vi "VoltageRatioInputStart.vi"(0 "Device Info":T1={"Serial Number"=-1, "Channel"=0, "Port"=0}, 1 "Data Interval":i32=-1, 2 "Change Trigger":dbl, 3 "Sesnor Type":u32(ring) caption="Sensor Type" items=["SENSOR_TYPE_VOLTAGERATIO"=0, "SENSOR_TYPE_1101_SHARP_2D120X"=11011, "SENSOR_TYPE_1101_SHARP_2Y0A21"=11012, "SENSOR_TYPE_1101_SHARP_2Y0A02"=11013, "SENSOR_TYPE_1102"=11020, "SENSOR_TYPE_1103"=11030, "SENSOR_TYPE_1104"=11040, "SENSOR_TYPE_1105"=11050, "SENSOR_TYPE_1106"=11060, "SENSOR_TYPE_1107"=11070, "SENSOR_TYPE_1108"=11080, "SENSOR_TYPE_1109"=11090, "SENSOR_TYPE_1110"=11100, "SENSOR_TYPE_1111"=11110, "SENSOR_TYPE_1112"=11120, "SENSOR_TYPE_1113"=11130, "SENSOR_TYPE_1115"=11150, "SENSOR_TYPE_1116"=11160, "SENSOR_TYPE_1118_AC"=11181, "SENSOR_TYPE_1118_DC"=11182, "SENSOR_TYPE_1119_AC"=11191, "SENSOR_TYPE_1119_DC"=11192, "SENSOR_TYPE_1120"=11200, "SENSOR_TYPE_1121"=11210, "SENSOR_TYPE_1122_AC"=11221, "SENSOR_TYPE_1122_DC"=11222, "SENSOR_TYPE_1124"=11240, "SENSOR_TYPE_1125_HUMIDITY"=11251, "SENSOR_TYPE_1125_TEMPERATURE"=11252, "SENSOR_TYPE_1126"=11260, "SENSOR_TYPE_1128"=11280, "SENSOR_TYPE_1129"=11290, "SENSOR_TYPE_1131"=11310, "SENSOR_TYPE_1134"=11340, "SENSOR_TYPE_1136"=11360, "SENSOR_TYPE_1137"=11370, "SENSOR_TYPE_1138"=11380, "SENSOR_TYPE_1139"=11390, "SENSOR_TYPE_1140"=11400, "SENSOR_TYPE_1141"=11410, "SENSOR_TYPE_1146"=11460, "SENSOR_TYPE_3120"=31200, "SENSOR_TYPE_3121"=31210, "SENSOR_TYPE_3122"=31220, "SENSOR_TYPE_3123"=31230, "SENSOR_TYPE_3130"=31300, "SENSOR_TYPE_3520"=35200, "SENSOR_TYPE_3521"=35210, "SENSOR_TYPE_3522"=35220], 5 "IsHubPort":bool, 7 "Bridge Enabled":bool=TRUE, 9 "Bridge Gain":u32(ring)=8 items=["BRIDGE_GAIN_1"=1, "BRIDGE_GAIN_2"=2, "BRIDGE_GAIN_4"=3, "BRIDGE_GAIN_8"=4, "BRIDGE_GAIN_16"=5, "BRIDGE_GAIN_32"=6, "BRIDGE_GAIN_64"=7, "BRIDGE_GAIN_128"=8], 11 "error in (no error)":errorcluster, 12 "Connection":u16(ring) items=["No Preference", "Remote", "Local"], 13 "Timeout (mSec)":i32=5000) -> (4 "Phidget ID":u64, 6 "Serial Number Return":i32, 10 "Attached?":bool, 15 "error out":errorcluster)   [LabVIEW 2012, in "Phidget Voltage Ratio Input.lvlib"]
doc: "${VoltageRatioInput:StartHeader}"
uses:
  <instrlib>/Phidgets/Phidget Voltage Ratio Input/Phidget Voltage Ratio Input.lvlib
  <instrlib>/Phidgets/Phidget Common/Phidget Common.lvlib
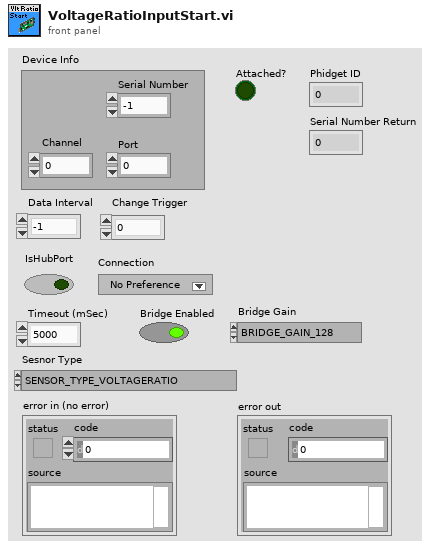
[diagram p1: front panel]
types:
  T1 = cluster{"Serial Number":i32, "Channel":i32, "Port":i32}
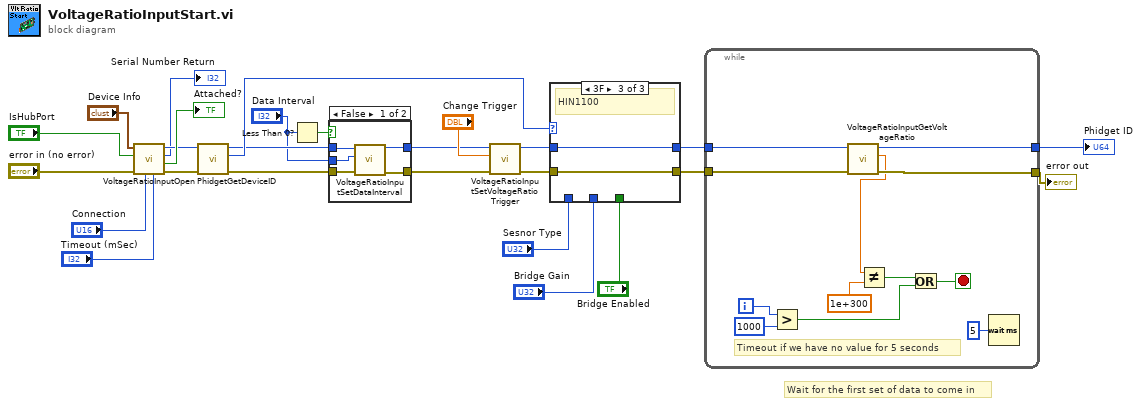
[diagram p0: block diagram]
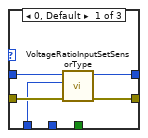
[diagram p3: hidden frame]
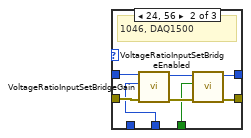
[diagram p4: hidden frame]
diagram:
  # "Wait for the first set of data to come in"
  n1 = call <instrlib>:"VoltageRatioInputOpen.vi"("Timeout (mSec)"="Timeout (mSec)", "Connection"="Connection", "error in"="error in (no error)", "IsHubPort"="IsHubPort", "Device Info"="Device Info") -> ("error out"=w23:errorcluster, "Attached?"=→"Attached?":bool, "Serial Number Return"=→"Serial Number Return":i32, "Phidget ID"=w22:u64)  [unwired: 3 in]
  n2 = call <instrlib>:"PhidgetGetDeviceID.vi"("error in (no error)"=w23, "Device In"=w22) -> ("error out"=w5:errorcluster, "Devie IDs"=w10:u32, "Device Out"=w4:u64)  [unwired: 6 in]
  n3 = Less Than 0?(x="Data Interval") -> (x < 0?=w6:bool)
  n4 = case shown="False" w6 {
    tunnel: w4 -> [w31 w33]
    tunnel: w5 -> [w30 w32]
    tunnel: [w28 w33] -> w2
    tunnel: [w29 w32] -> w1
    tunnel: "Data Interval" -> [w27 _]
    frame False {
      n5 = call <instrlib>:"VoltageRatioInputSetDataInterval.vi"("error in (no error)"=w30, "Interval"=w27, "Device In"=w31) -> ("error out"=w29:errorcluster, "Device Out"=w28:u64)  [unwired: 6 in]
    }
    frame True {
    }
  }
  n6 = call <instrlib>:"VoltageRatioInputSetVoltageRatioTrigger.vi"("error in (no error)"=w1, "Trigger"="Change Trigger", "Device In"=w2) -> ("error out"=w14:errorcluster, "Device Out"=w13:u64)  [unwired: 6 in]
  n7 = case shown="3F" w10 {
    tunnel: w14 -> [w38 w42 w47]
    tunnel: w13 -> [w37 w41 w48]
    tunnel: [w36 w43 w47] -> w12
    tunnel: [w35 w44 w48] -> w11
    tunnel: "Sesnor Type" -> [w34 _ _]
    tunnel: "Bridge Gain" -> [_ w40 _]
    tunnel: "Bridge Enabled" -> [_ w39 _]
    frame 0, Default {
      n8 = call <instrlib>:"VoltageRatioInputSetSensorType.vi"("error in (no error)"=w38, "Sesnor Type"=w34, "Device In"=w37) -> ("error out"=w36:errorcluster, "Device Out"=w35:u64)  [unwired: 6 in]
    }
    frame 24, 56 {
      # "1046, DAQ1500"
      n9 = call <instrlib>:"VoltageRatioInputSetBridgeGain.vi"("error in (no error)"=w42, "Bridge Gain"=w40, "Device In"=w41) -> ("error out"=w45:errorcluster, "Device Out"=w46:u64)  [unwired: 6 in]
      n10 = call <instrlib>:"VoltageRatioInputSetBridgeEnabled.vi"("error in (no error)"=w45, "Bridge Enabled"=w39, "Device In"=w46) -> ("error out"=w43:errorcluster, "Device Out"=w44:u64)  [unwired: 6 in]
    }
    frame 63 {
      # "HIN1100"
    }
  }
  n11 = while {
    tunnel: w11 -> [w58]
    tunnel: w12 -> [w57]
    tunnel: [w55] -> w21
    tunnel: [w56] -> w25
    i -> [w53]
    stop <- w50 stop-if-true
    # "Timeout if we have no value for 5 seconds"
    n12 = Greater?(x=w53, y=1000) -> (0:w51:bool)
    n13 = call <instrlib>:"VoltageRatioInputGetVoltageRatio.vi"("error in (no error)"=w57, "Device In"=w58) -> ("error out"=w56:errorcluster, "Voltage Ratio"=w49:dbl, "Device Out"=w55:u64)  [unwired: 6 in]
    n14 = Not Equal?(x=w49, y=1e+300) -> (x != y?=w52:bool)
    n15 = Or(x=w52, y=w51) -> (x .or. y?=w50:bool)
    n16 = Wait (ms)(milliseconds to wait=u32 5) -> ()  [unwired: 1 out]
  }
  "error out" <- w25
  "Phidget ID" <- w21
